vi "log.vi"() -> ()   [LabVIEW 2020]
uses:
  <vilib>/Utility/file.llb/Read Delimited Spreadsheet (string).vi
panel:
  out "all rows 2":string[](array[string])
  out "all rows":string[][](array[string])
  out "login status":string
  in  "Log in confirm":bool
  in  "请输入账号":string caption="Please enter your account:"
  in  "请输入密码":string caption="Please enter your password:"
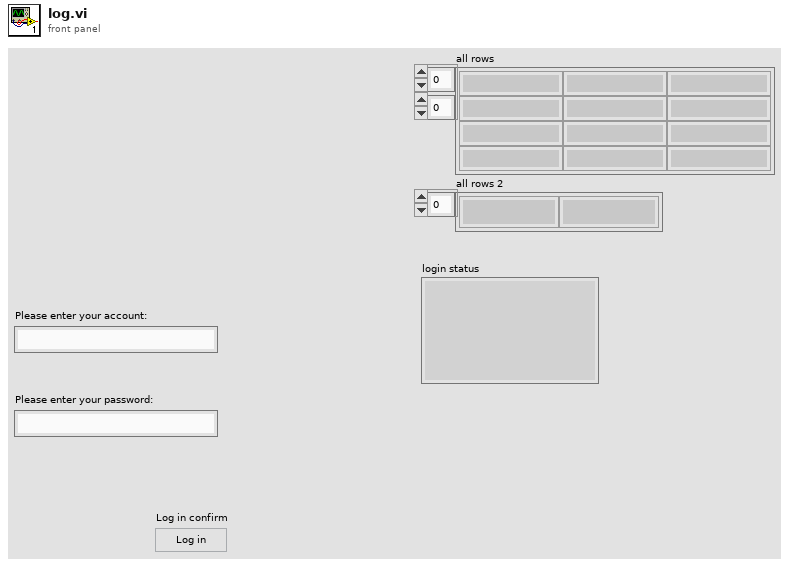
[diagram p1: front panel]
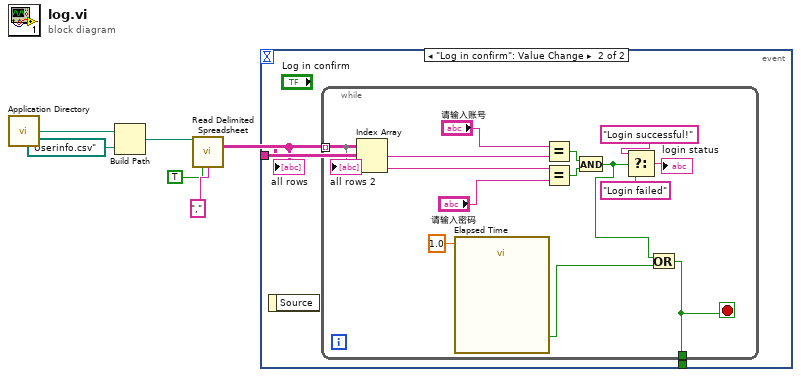
[diagram p0: block diagram]
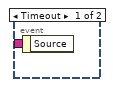
[diagram p2: hidden frame]
diagram:
  n1 = call <vilib>:"Application Directory.vi"() -> ("Application Directory"=w6:path)
  n2 = Build Path(base path=w6, name or relative path=path "Userinfo.csv") -> (appended path=w3:path)
  n3 = call-poly <vilib>:"Read Delimited Spreadsheet.vi"("file path (dialog if empty)"=w3, "transpose? (F)"=TRUE, "delimiter (\\t)"="," ("delimiter (\\t)")) -> ("all rows"=w1:string[][])  [unwired: 7 in, 5 out]
  n4 = event shown="[1] \"Log in confirm\": Value Change" {
    selector: _ -> [_ _]
    dyn-events: _ -> [_ _]
    timeout: _ -> [_ _]
    tunnel: w1 -> [_ w8]
    tunnel: [_ w7] -> _
    event Timeout {
      n5 = event-data() -> ()  [unwired: 1 in, 1 out]
    }
    event "Log in confirm": Value Change {
      n6 = event-data() -> ()  [unwired: 1 in, 1 out]
      n7 = while {
        tunnel: w8 -> [w22] mode=indexing
        tunnel: [w9] -> w7
        stop <- w9 stop-if-true
        n8 = Index Array(array=w22) -> (element #1=w15:string, element #2=w14:string)  [unwired: 2 in]
        n9 = call "Elapsed Time"("Time Target (s)"=1.0) -> ("Time has Elapsed"=w11:bool)  [unwired: 11 in, 7 out]
        n10 = Equal?(x="请输入账号", y=w15) -> (x = y?=w19:bool)
        n11 = Equal?(x=w14, y="请输入密码") -> (x = y?=w18:bool)
        n12 = And(x=w19, y=w18) -> (x .and. y?=w10:bool)
        n13 = Select(t="Login successful!", s=w10, f="Login failed") -> (s? t:f=→"login status":string)
        n14 = Or(x=w10, y=w11) -> (x .or. y?=w9:bool)
        "all rows 2" <- w22
      }
      "all rows" <- w8
    }
  }
